vi "Write AllowUserToAddRows.vi"(8 "error in (no error)":errorcluster, 10 "AllowUserToAddRows":bool, 11 "DataGridView in":refnum<class "DataGridView.lvclass">) -> (0 "error out":errorcluster, 3 "DataGridView out":refnum<class "DataGridView.lvclass">)   [LabVIEW 2014, in "DataGridView.lvclass"]
uses:
  DataGridView.lvclass
  DataGridView.lvclass/DataGridView.ctl
  System.Windows.Forms
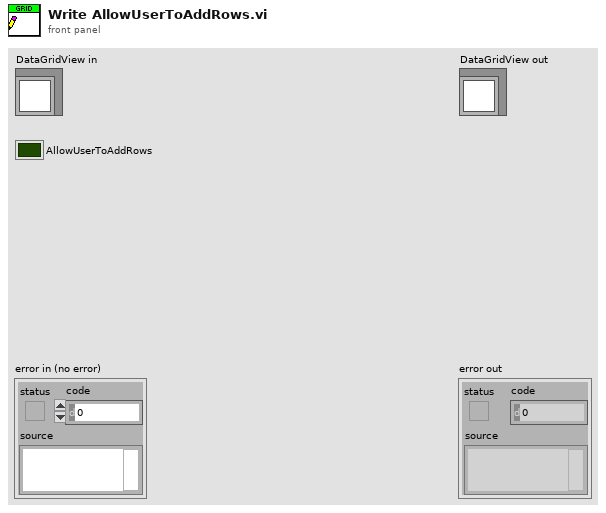
[diagram p1: front panel]
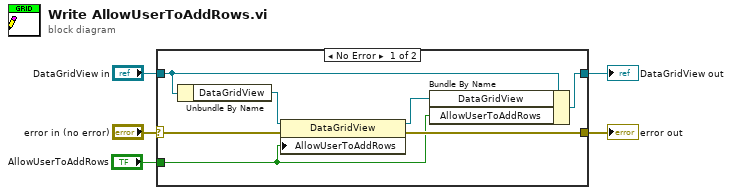
[diagram p0: block diagram]
diagram:
  n1 = case shown="No Error" "error in (no error)" {
    selector: "error in (no error)" -> [w12 w13]
    tunnel: [w11 w13] -> w4
    tunnel: [w8 w14] -> w2
    tunnel: "DataGridView in" -> [w6 w14]
    tunnel: "AllowUserToAddRows" -> [w7 _]
    frame No Error {
      n2 = Unbundle By Name(w6) -> ("DataGridView"=w10:refnum<k24>)
      n3 = property class="DataGridView"(reference=w10, error in=w12, "AllowUserToAddRows"=w7) -> (reference out=w9:refnum<k24>, error out=w11:errorcluster)
      n4 = Bundle By Name(cluster=w6, "DataGridView"=w9, "AllowUserToAddRows"=w7) -> (w8:refnum<class "DataGridView.lvclass">)
    }
    frame Error {
    }
  }
  "error out" <- w4
  "DataGridView out" <- w2
